vi "range distances (SubVI).vi"(8 "mid_to_targ_dist":sgl, 9 "Set#1 Separation":sgl, 10 "Barrel to Screen":sgl) -> (0 "scr#2 / target":string, 1 "Set#1 Separation":string, 2 "muzzle / scr#1":string, 3 "muzzle / target":string, 4 "mid_to_targ_dist":string)   [LabVIEW 2015]
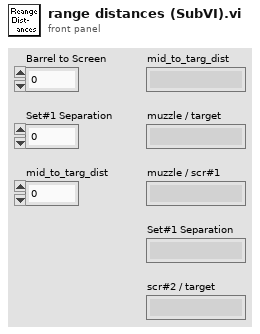
[diagram p1: front panel]
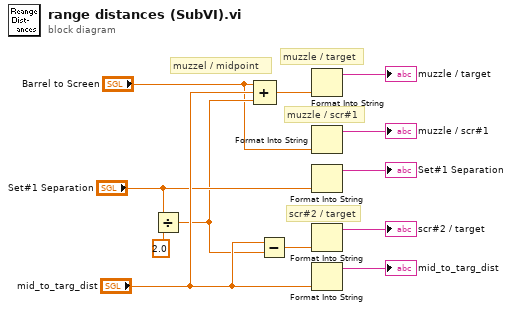
[diagram p0: block diagram]
diagram:
  # "muzzel / midpoint"
  # "muzzle / scr#1"
  # "muzzle / target"
  # "scr#2 / target"
  n1 = Divide(x="Set#1 Separation", y=sgl 2.0) -> (x/y=w2:sgl)
  n2 = Compound Arithmetic op=ADD("Barrel to Screen", "mid_to_targ_dist", w2) -> (w8:sgl)
  n3 = Subtract(x="mid_to_targ_dist", y=w2) -> (x-y=w11:sgl)
  n4 = Format Into String(w8) -> (resulting string=→"muzzle / target":string)  [unwired: 3 in, 1 out]
  n5 = Format Into String("Barrel to Screen") -> (resulting string=→"muzzle / scr#1":string)  [unwired: 3 in, 1 out]
  n6 = Format Into String("Set#1 Separation") -> (resulting string=→"Set#1 Separation":string)  [unwired: 3 in, 1 out]
  n7 = Format Into String(w11) -> (resulting string=→"scr#2 / target":string)  [unwired: 3 in, 1 out]
  n8 = Format Into String("mid_to_targ_dist") -> (resulting string=→"mid_to_targ_dist":string)  [unwired: 3 in, 1 out]
